vi "Open Audio File Write (WAV).vi"(8 "error in (no error)":errorcluster, 9 "Codec Specific Info":T1={"Container Format"=enum."RIFF", "Data Format"=1} {"Data Format" items=["PCM"=1, "ADPCM"=2, "IEEE Float"=3]}, 10 "Audio File Info":T4={"Sample Rate (Hz)"=44100, "Channels"=2, "Bit Depth"=16}, 11 "Path":path) -> (0 "error out":errorcluster, 3 "Audio File Refnum":refnum<file>)   [LabVIEW 2020, in "G-Audio.lvlib"]
doc: "Create or replace an audio file and initialize the WAV encoder for writing."
uses:
  G-Audio.lvlib
  Controls/Audio File Info.ctl
  Controls/WAV Codec Specific Info.ctl
  Controls/WAV Container Format.ctl
  Controls/WAV Data Format.ctl
  <vilib>/Utility/error.llb/Error Cluster From Error Code.vi
  lib/g_audio_x86.dll
  lib/g_audio_x64.dll
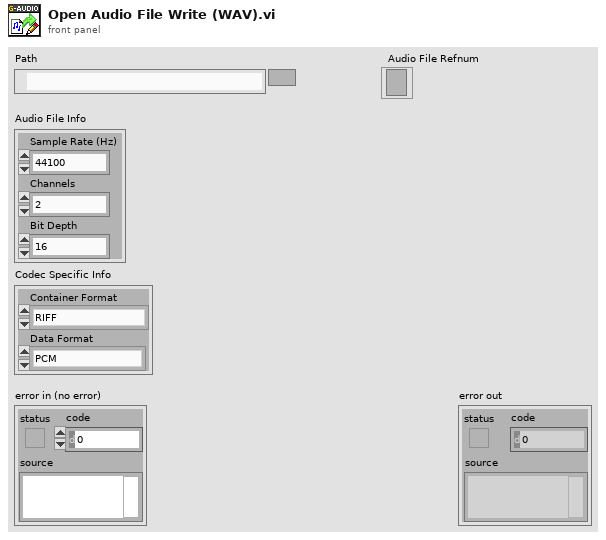
[diagram p1: front panel]
types:
  T1 = typedef "G-Audio.lvlib/WAV Codec Specific Info.ctl" = cluster{"Container Format":T2, "Data Format":T3}
  T2 = typedef "G-Audio.lvlib/WAV Container Format.ctl" = enum32{"RIFF", "Wave64"}
  T3 = typedef "G-Audio.lvlib/WAV Data Format.ctl" = u32
  T4 = typedef "G-Audio.lvlib/Audio File Info.ctl" = cluster{"Sample Rate (Hz)":u32, "Channels":u32, "Bit Depth":u32}
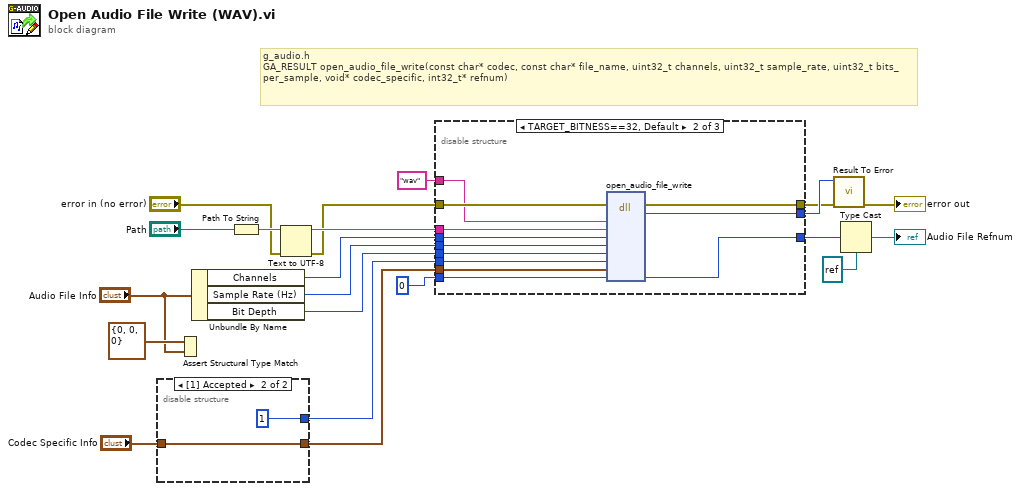
[diagram p0: block diagram]
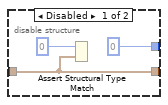
[diagram p2: hidden frame]
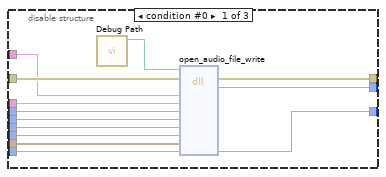
[diagram p3: hidden frame]
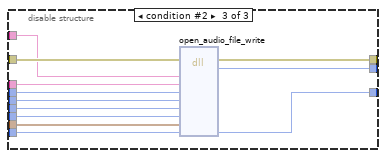
[diagram p4: hidden frame]
diagram:
  # "g_audio.h\nGA_RESULT open_audio_file_write(const char* codec, const char* file_name, uint32_t channels, uint32_t sample_rate, uint32_t bits_per_sample, void* codec_specific, int32_t* refnum)"
  n1 = disable-structure shown="[1] Accepted" {
    disable-tunnel: "Codec Specific Info" -> [w22 w25]
    disable-tunnel: [0 1] -> w5
    disable-tunnel: [w22 w25] -> w4
    frame Disabled {
      n2 = Assert Structural Type Match(0:w22, 1:0) -> ()
    }
    frame Enabled {
    }
  }
  n3 = Assert Structural Type Match(0:"Audio File Info", 1:T4 {"Sample Rate (Hz)"=0, "Channels"=0, "Bit Depth"=0} ("Audio File Info 2")) -> ()
  n4 = Unbundle By Name("Audio File Info") -> ("Channels"=w11:u32, "Sample Rate (Hz)"=w10:u32, "Bit Depth"=w9:u32)
  n5 = Path To String(path="Path") -> (string=w14:string)
  n6 = Text to UTF-8(8:"error in (no error)", 11:w14) -> (0:w12:errorcluster, 3:w13:string)  [unwired: 1 in]
  n7 = disable-structure shown="TARGET_BITNESS==32, Default" {
    disable-tunnel: w12 -> [w39 w51 w63]
    disable-tunnel: w13 -> [w37 w49 w61]
    disable-tunnel: [w38 w50 w62] -> w16
    disable-tunnel: 0 ("num_samples") -> [w35 w47 w59]
    disable-tunnel: "wav" ("Codec Out") -> [w36 w48 w60]
    disable-tunnel: [w34 w46 w58] -> w19
    disable-tunnel: [w33 w45 w57] -> w17
    disable-tunnel: w11 -> [w31 w44 w56]
    disable-tunnel: w10 -> [w30 w43 w55]
    disable-tunnel: w9 -> [w29 w42 w54]
    disable-tunnel: w4 -> [w28 w41 w53]
    disable-tunnel: w5 -> [w27 w40 w52]
    frame condition #0 {
      n8 = call "Debug Path.vi"() -> ("Debug Path"=w32:path)  [unwired: 11 in]
      n9 = dll-call lib="?" fn="open_audio_file_write"(path in=w32, error in=w39, "codec"=w36, "file_name"=w37, "channels"=w31, "sample_rate"=w30, "bits_per_sample"=w29, "has_specific_info"=w27, "codec_specific"=w28, "refnum"=w35) -> (error out=w38:errorcluster, "result"=w33:i32, "refnum"=w34:i32)  [unwired: 8 in, 1 out]
    }
    frame condition #1 (active) {
      n10 = dll-call lib="C:/github/dataflowg/g-audio/src/LabVIEW/G-Audio/lib/g_audio_x86.*" fn="open_audio_file_write"(error in=w51, "codec"=w48, "file_name"=w49, "channels"=w44, "sample_rate"=w43, "bits_per_sample"=w42, "has_specific_info"=w40, "codec_specific"=w41, "refnum"=w47) -> (error out=w50:errorcluster, "result"=w45:i32, "refnum"=w46:i32)  [unwired: 9 in, 1 out]
    }
    frame condition #2 {
      n11 = dll-call lib="C:/github/dataflowg/g-audio/src/LabVIEW/G-Audio/lib/g_audio_x64.*" fn="open_audio_file_write"(error in=w63, "codec"=w60, "file_name"=w61, "channels"=w56, "sample_rate"=w55, "bits_per_sample"=w54, "has_specific_info"=w52, "codec_specific"=w53, "refnum"=w59) -> (error out=w62:errorcluster, "result"=w57:i32, "refnum"=w58:i32)  [unwired: 9 in, 1 out]
    }
  }
  n12 = call "Result To Error.vi"("error in (no error)"=w16, "Result Code"=w17) -> ("error out"=→"error out":errorcluster)  [unwired: 9 in]
  n13 = Type Cast(type=refnum<file> refnum ("Audio File Refnum"), x=w19) -> (*(type *) &x=→"Audio File Refnum":refnum<file>)
